vi "LJM_ByteArrayToFLOAT32.vi"(1 "Byte Array":u8[](array[numeric])) -> (0 "Float":sgl format="%.6f")   [LabVIEW 2020]
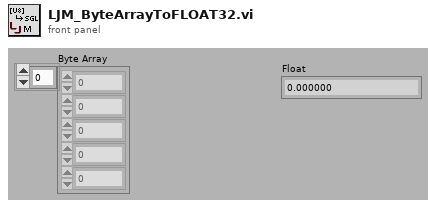
[diagram p1: front panel]
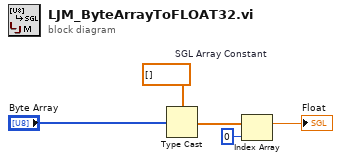
[diagram p0: block diagram]
diagram:
  w5 = sgl[] []  # SGL Array Constant
  n1 = Type Cast(type=w5, x="Byte Array") -> (*(type *) &x=w2:sgl[])
  n2 = Index Array(array=w2, index=0 ("Index")) -> (element=→"Float":sgl)
